vi "Read FF buffers.vi"(8 "error in (no error)":errorcluster, 10 "Force":bool, 11 "FpgaRef5785 in":refnum<class "FpgaRef5782.lvclass">) -> (0 "error out":errorcluster, 2 "Scaled":dbl[][](array[numeric]), 3 "FpgaRef5785 out":refnum<class "FpgaRef5782.lvclass">)   [LabVIEW 2018, in "FpgaRef5782.lvclass"]
uses:
  FpgaRef5782.lvclass
  FpgaRef5782.lvclass/FpgaRef5782.ctl
  <vilib>/Utility/error.llb/Error Cluster From Error Code.vi
  <vilib>/rvi/errors/niLvFpgaAdjustHostInterfaceError.vi
  <vilib>/rvi/interface/nirviMethod/nirviMethod.xnode
  5782 FPGA ref.ctl
  <vilib>/rvi/interface/nirviReadWriteControl/nirviReadWriteControl.xnode
  NiFpgaLv.dll
  <vilib>/rvi/interface/Simulation/niFpgaSimulationCallBeginRW.vi
  <vilib>/FPGAPlugInAG/Dynamic/niLvFpga_ReadFifo_Dynamic.vi
  <vilib>/rvi/errors/niLvFpgaMergeErrorWithErrorCode.vi
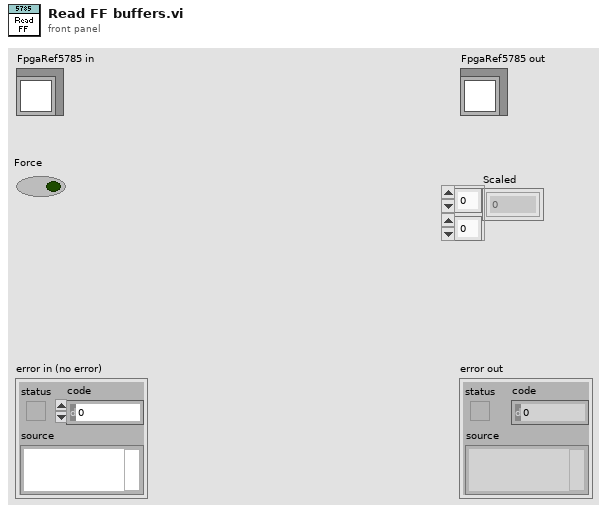
[diagram p1: front panel]
types:
  T1 = typedef "5782 FPGA ref.ctl" = refnum<k20>
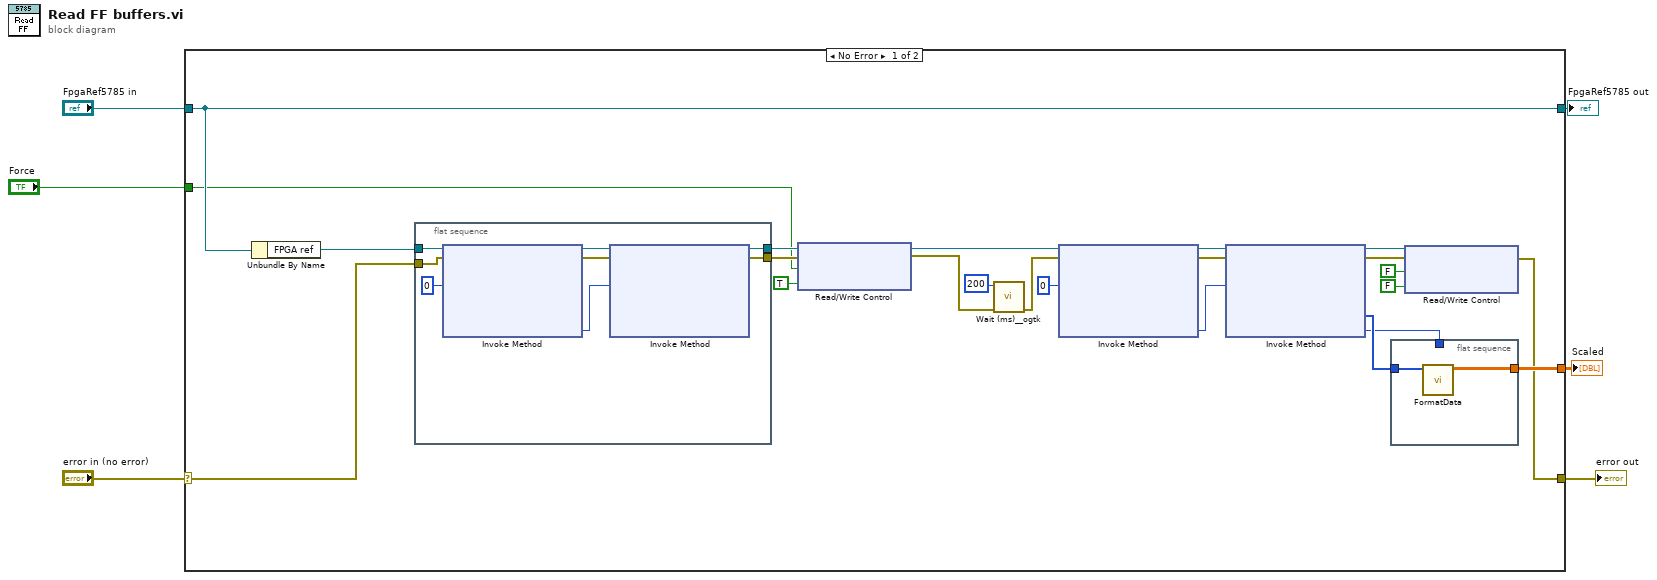
[diagram p0: block diagram]
diagram:
  n1 = case shown="No Error" "error in (no error)" {
    selector: "error in (no error)" -> [w12 w41]
    tunnel: [w11 w41] -> w5
    tunnel: [w15 w40] -> w3
    tunnel: "FpgaRef5785 in" -> [w15 w40]
    tunnel: [w13 _] -> w2
    tunnel: "Force" -> [w10 _]
    frame No Error {
      n2 = Unbundle By Name(w15) -> ("FPGA ref"=w14:T1)
      n3 = flat-sequence {
        tunnel: w14 -> [w35]
        tunnel: [w33] -> w29
        tunnel: [w31] -> w18
        tunnel: w12 -> [w30]
        frame #0 {
          n4 = xnode "Invoke Method"("FPGA VI Reference In"=w35, "error in"=w30, "Number of Elements"=u32 0) -> ("FPGA VI Reference Out"=w34:T1, "error out"=w32:errorcluster, "Elements Remaining"=w36:u32)  [unwired: 1 in, 1 out]
          n5 = xnode "Invoke Method"("FPGA VI Reference In"=w34, "error in"=w32, "Number of Elements"=w36) -> ("FPGA VI Reference Out"=w33:T1, "error out"=w31:errorcluster)  [unwired: 1 in, 2 out]
        }
      }
      n6 = xnode "Read/Write Control"("FPGA VI Reference In"=w29, "error in"=w18, "FF buffers manual"=w10, "Load FF"=TRUE) -> ("FPGA VI Reference Out"=w22:T1, "error out"=w27:errorcluster)
      n7 = call <userlib>:"Wait (ms)__ogtk.vi"("error in (no error)"=w27, "milliseconds to wait"=u32 200) -> ("error out"=w21:errorcluster)  [unwired: 8 in, 1 out]
      n8 = xnode "Invoke Method"("FPGA VI Reference In"=w22, "error in"=w21, "Number of Elements"=u32 0) -> ("FPGA VI Reference Out"=w25:T1, "error out"=w17:errorcluster, "Elements Remaining"=w24:u32)  [unwired: 1 in, 1 out]
      n9 = xnode "Invoke Method"("FPGA VI Reference In"=w25, "error in"=w17, "Number of Elements"=w24) -> ("FPGA VI Reference Out"=w19:T1, "error out"=w16:errorcluster, "Data"=w9:u64[], "Elements Remaining"=w7:u32)  [unwired: 1 in]
      n10 = flat-sequence {
        tunnel: w9 -> [w39]
        tunnel: [w38] -> w13
        tunnel: w7 -> [_]
        frame #0 {
          n11 = call "FormatData.vi"("Raw data"=w39) -> ("Scaled"=w38:dbl[][])  [unwired: 10 in]
        }
      }
      n12 = xnode "Read/Write Control"("FPGA VI Reference In"=w19, "error in"=w16, "Load FF"=FALSE, "FF buffers manual"=FALSE) -> ("error out"=w11:errorcluster)  [unwired: 1 out]
    }
    frame Error {
    }
  }
  "error out" <- w5
  "FpgaRef5785 out" <- w3
  "Scaled" <- w2
